vi "Process Interfaces.vi"(8 "error in (no error)":errorcluster {"code" format="Error %.0f"}, 10 "Interfaces":refnum<class "Interface Documenation.lvclass">[](array[class]), 11 "VIDoc Printer In":refnum<class "VIDoc Printer.lvclass">) -> (0 "error out":errorcluster {"code" format="Error %.0f"}, 3 "VIDoc Printer Out":refnum<class "VIDoc Printer.lvclass">)   [LabVIEW 2023, in "VIDoc Printer.lvlib" / "VIDoc Printer.lvclass"]
uses:
  VIDoc Printer.lvclass
  VIDoc Printer.lvclass/VIDoc Printer.ctl
  Parsing/Interface Documenation/Interface Documenation.lvclass
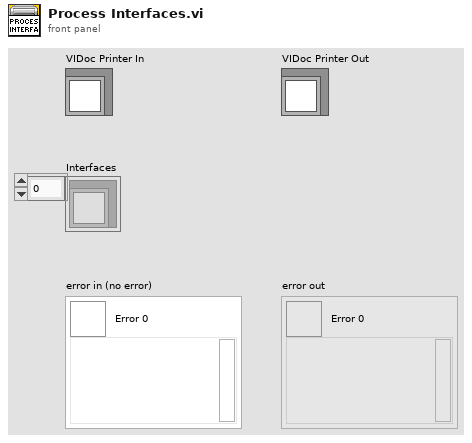
[diagram p1: front panel]
types:
  T1 = typedef "VIDoc Printer.lvlib/VIDoc Printer.lvclass/Process Interfaces Enum.ctl" = enum16{"Headers", "Memory", "By List", "Description", "Inheritance", "Inheritance Parent Interfaces", "Inheritance Friends", "Methods", "Controls"}
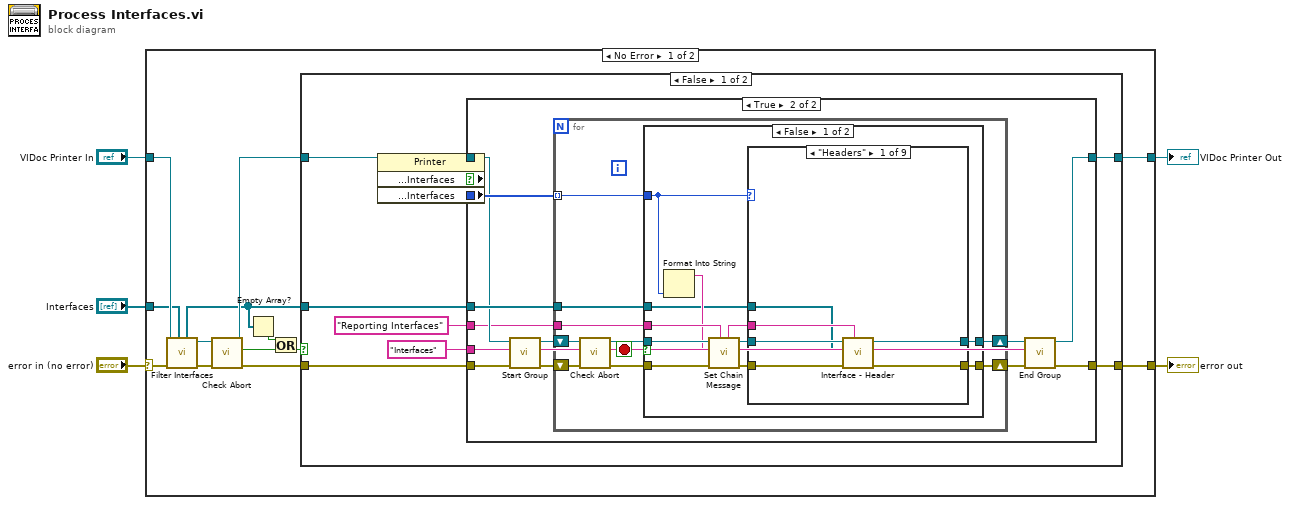
[diagram p0: block diagram]
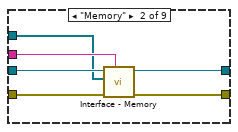
[diagram p3: hidden frame]
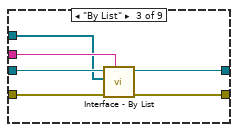
[diagram p4: hidden frame]
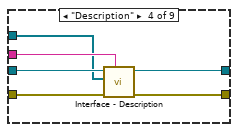
[diagram p5: hidden frame]
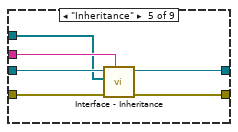
[diagram p6: hidden frame]
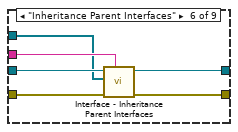
[diagram p7: hidden frame]
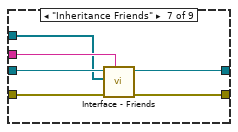
[diagram p8: hidden frame]
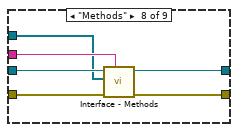
[diagram p9: hidden frame]
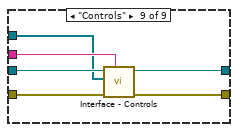
[diagram p10: hidden frame]
diagram:
  n1 = case shown="No Error" "error in (no error)" {
    selector: "error in (no error)" -> [w18 w123]
    tunnel: [w14 w123] -> w2
    tunnel: [w13 w122] -> w1
    tunnel: "VIDoc Printer In" -> [w8 w122]
    tunnel: "Interfaces" -> [w6 _]
    frame No Error {
      n2 = call "Filter Interfaces.vi"("Interfaces"=w6, "error in (no error)"=w18, "VIDoc Printer In"=w8) -> ("error out"=w10:errorcluster, "VIDoc Printer Out"=w9:refnum<class "VIDoc Printer.lvclass">, "Filtered Interfaces"=w7:refnum<class "Interface Documenation.lvclass">[])  [unwired: 6 in]
      n3 = call "Check Abort.vi"("error in (no error)"=w10, "VIDoc Printer In"=w9) -> ("error out"=w17:errorcluster, "Abort?"=w15:bool, "VIDoc Printer Out"=w16:refnum<class "VIDoc Printer.lvclass">)  [unwired: 7 in]
      n4 = Empty Array?(array=w7) -> (empty?=w11:bool)
      n5 = Or(x=w11, y=w15) -> (x .or. y?=w12:bool)
      n6 = case shown="False" w12 {
        tunnel: w7 -> [w28 _]
        tunnel: w17 -> [w25 w121]
        tunnel: w16 -> [w26 w120]
        tunnel: [w23 w121] -> w14
        tunnel: [w24 w120] -> w13
        frame False {
          n7 = property class="Printer"(reference=w26) -> (reference out=w27:refnum<class "VIDoc Printer.lvclass">, "Properties:Settings:Enabled Sections:Interfaces"=w20:bool, "Properties:Process Lists:Interfaces"=w19:T1[])  [unwired: 1 in, 1 out]
          n8 = case shown="True" w20 {
            tunnel: w25 -> [w30 w40]
            tunnel: "Reporting Interfaces" ("Section") -> [_ w32]
            tunnel: [w30 w33] -> w23
            tunnel: w28 -> [_ w42]
            tunnel: w27 -> [w29 w37]
            tunnel: [w29 w34] -> w24
            tunnel: w19 -> [_ w41]
            tunnel: "Interfaces" ("Section") -> [_ w31]
            frame False {
            }
            frame True {
              n9 = call-dynamic "Start Group.vi"("error in (no error)"=w40, "Group"=w31, "VIDoc Printer In"=w37) -> ("error out"=w39:errorcluster, "VIDoc Printer Out"=w38:refnum<class "VIDoc Printer.lvclass">)  [unwired: 7 in]
              n10 = for {
                shift-right: [w50] -> w35
                shift-left: w39 -> [w52]
                tunnel: w32 -> [w46]
                tunnel: w42 -> [w45]
                shift-right: [w48] -> w36
                shift-left: w38 -> [w51]
                tunnel: w41 -> [w44] mode=indexing
                stop <- w43 stop-if-true
                n11 = call "Check Abort.vi"("error in (no error)"=w52, "VIDoc Printer In"=w51) -> ("error out"=w49:errorcluster, "Abort?"=w43:bool, "VIDoc Printer Out"=w47:refnum<class "VIDoc Printer.lvclass">)  [unwired: 7 in]
                n12 = case shown="False" w43 {
                  tunnel: [w63 w119] -> w50
                  tunnel: w49 -> [w60 w119]
                  tunnel: [w62 w118] -> w48
                  tunnel: w47 -> [w58 w118]
                  tunnel: w46 -> [w57 _]
                  tunnel: w45 -> [w54 _]
                  tunnel: w44 -> [w56 _]
                  frame False {
                    n13 = Format Into String(w56) -> (resulting string=w55:string)  [unwired: 3 in, 1 out]
                    n14 = call "Set Chain Message.vi"("Msg Chain"=w57, "error in (no error)"=w60, "New"=w55, "VIDoc Printer In"=w58) -> ("error out"=w61:errorcluster, "VIDoc Printer Out"=w59:refnum<class "VIDoc Printer.lvclass">, "Msg Chain out"=w53:string)  [unwired: 5 in]
                    n15 = case shown="\"Headers\"" w56 {
                      tunnel: w61 -> [w68 w74 w80 w86 w92 w98 w104 w110 w116]
                      tunnel: [w66 w72 w78 w84 w90 w96 w102 w108 w114] -> w63
                      tunnel: w59 -> [w69 w75 w81 w87 w93 w99 w105 w111 w117]
                      tunnel: [w67 w73 w79 w85 w91 w97 w103 w109 w115] -> w62
                      tunnel: w54 -> [w64 w70 w76 w82 w88 w94 w100 w106 w112]
                      tunnel: w53 -> [w65 w71 w77 w83 w89 w95 w101 w107 w113]
                      frame "Headers" {
                        n16 = call-dynamic "Interface - Header.vi"("Msg Chain"=w65, "error in (no error)"=w68, "Interfaces"=w64, "VIDoc Printer In"=w69) -> ("error out"=w66:errorcluster, "VIDoc Printer Out"=w67:refnum<class "VIDoc Printer.lvclass">)  [unwired: 6 in]
                      }
                      frame "Memory" {
                        n17 = call-dynamic "Interface - Memory.vi"("Msg Chain"=w71, "error in (no error)"=w74, "Interfaces"=w70, "VIDoc Printer In"=w75) -> ("error out"=w72:errorcluster, "VIDoc Printer Out"=w73:refnum<class "VIDoc Printer.lvclass">)  [unwired: 6 in]
                      }
                      frame "By List" {
                        n18 = call-dynamic "Interface - By List.vi"("Msg Chain"=w77, "error in (no error)"=w80, "Interfaces"=w76, "VIDoc Printer In"=w81) -> ("error out"=w78:errorcluster, "VIDoc Printer Out"=w79:refnum<class "VIDoc Printer.lvclass">)  [unwired: 6 in]
                      }
                      frame "Description" {
                        n19 = call-dynamic "Interface - Description.vi"("Msg Chain"=w83, "error in (no error)"=w86, "Interfaces"=w82, "VIDoc Printer In"=w87) -> ("error out"=w84:errorcluster, "VIDoc Printer Out"=w85:refnum<class "VIDoc Printer.lvclass">)  [unwired: 6 in]
                      }
                      frame "Inheritance" {
                        n20 = call-dynamic "Interface - Inheritance.vi"("Msg Chain"=w89, "error in (no error)"=w92, "Interfaces"=w88, "VIDoc Printer In"=w93) -> ("error out"=w90:errorcluster, "VIDoc Printer Out"=w91:refnum<class "VIDoc Printer.lvclass">)  [unwired: 6 in]
                      }
                      frame "Inheritance Parent Interfaces" {
                        n21 = call-dynamic "Interface - Inheritance Parent Interfaces.vi"("Msg Chain"=w95, "error in (no error)"=w98, "Interfaces"=w94, "VIDoc Printer In"=w99) -> ("error out"=w96:errorcluster, "VIDoc Printer Out"=w97:refnum<class "VIDoc Printer.lvclass">)  [unwired: 6 in]
                      }
                      frame "Inheritance Friends" {
                        n22 = call-dynamic "Interface - Friends.vi"("Msg Chain"=w101, "error in (no error)"=w104, "Interfaces"=w100, "VIDoc Printer In"=w105) -> ("error out"=w102:errorcluster, "VIDoc Printer Out"=w103:refnum<class "VIDoc Printer.lvclass">)  [unwired: 6 in]
                      }
                      frame "Methods" {
                        n23 = call-dynamic "Interface - Methods.vi"("Msg Chain"=w107, "error in (no error)"=w110, "Interfaces"=w106, "VIDoc Printer In"=w111) -> ("error out"=w108:errorcluster, "VIDoc Printer Out"=w109:refnum<class "VIDoc Printer.lvclass">)  [unwired: 6 in]
                      }
                      frame "Controls" {
                        n24 = call-dynamic "Interface - Controls.vi"("Msg Chain"=w113, "error in (no error)"=w116, "Interfaces"=w112, "VIDoc Printer In"=w117) -> ("error out"=w114:errorcluster, "VIDoc Printer Out"=w115:refnum<class "VIDoc Printer.lvclass">)  [unwired: 6 in]
                      }
                    }
                  }
                  frame True {
                  }
                }
              }
              n25 = call-dynamic "End Group.vi"("error in (no error)"=w35, "Group"=w31, "VIDoc Printer In"=w36) -> ("error out"=w33:errorcluster, "VIDoc Printer Out"=w34:refnum<class "VIDoc Printer.lvclass">)  [unwired: 7 in]
            }
          }
        }
        frame True {
        }
      }
    }
    frame Error {
    }
  }
  "error out" <- w2
  "VIDoc Printer Out" <- w1
